vi "Handle Click on Graph.vi"(6 "PlatMods":T1, 7 "Button":u16, 8 "error in (no error)":errorcluster, 9 "Mods":cluster{"Double Click":bool, "Menu Key":bool}, 10 "Coords":T2, 11 "GarphView in":refnum<class "GarphView.lvclass">) -> (0 "error out":errorcluster, 3 "GarphView out":refnum<class "GarphView.lvclass">)   [LabVIEW 2020, in "GarphView.lvlib" / "GarphView.lvclass"]
uses:
  GarphView.lvclass
  GarphView.lvclass/GarphView.ctl
  <vilib>/Utility/miscctls.llb/LVPoint32TypeDef.ctl
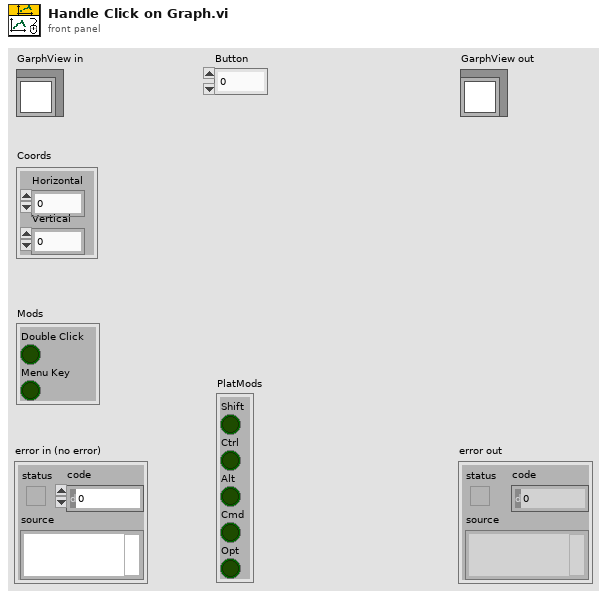
[diagram p1: front panel]
types:
  T1 = cluster{"Shift":bool, "Ctrl":bool, "Alt":bool, "Cmd":bool, "Opt":bool}
  T2 = typedef "LVPoint32TypeDef.ctl" = cluster{"Horizontal":i32, "Vertical":i32}
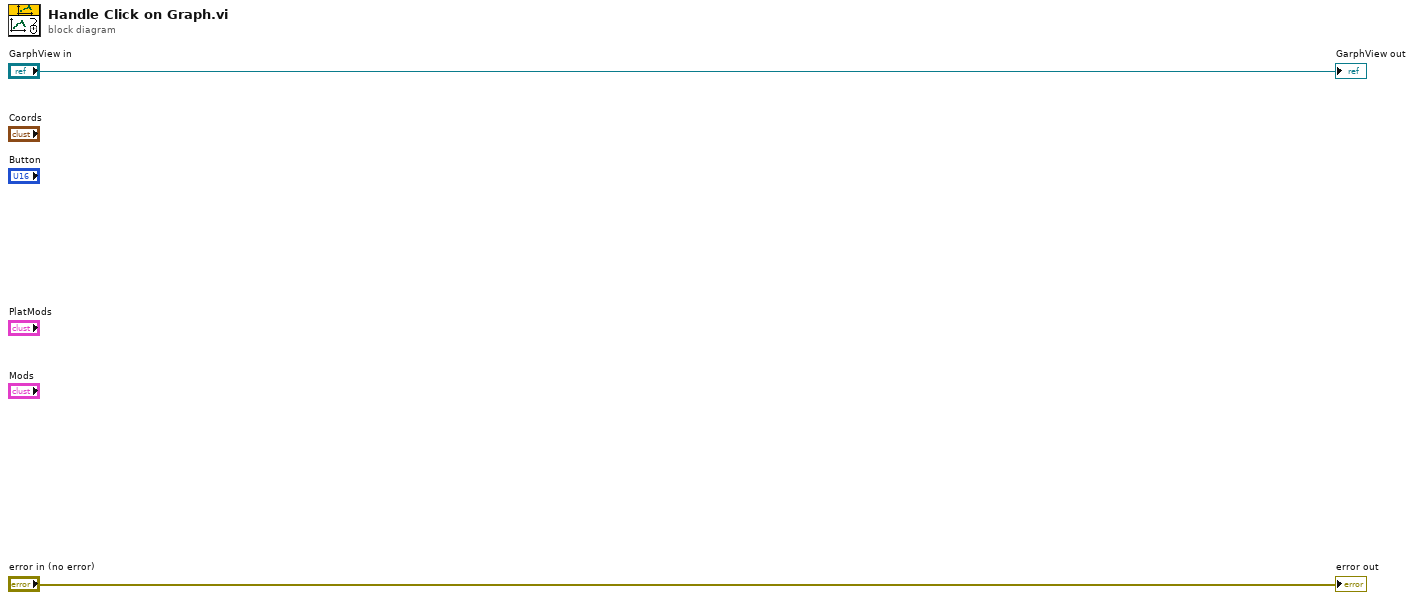
[diagram p0: block diagram]
diagram:
  "error out" <- "error in (no error)"
  "GarphView out" <- "GarphView in"
